vi "Enum from Ring String.vi"(8 "String to Match":string, 9 "Ring Strings []":string[](array[string]), 11 "Ring StringsAndValues[]":T1) -> (0 "error out":errorcluster, 3 "Enum Value":i32)   [LabVIEW 2024]
uses:
  <vilib>/Utility/miscctls.llb/LVStringsAndValuesArrayTypeDef_I32.ctl
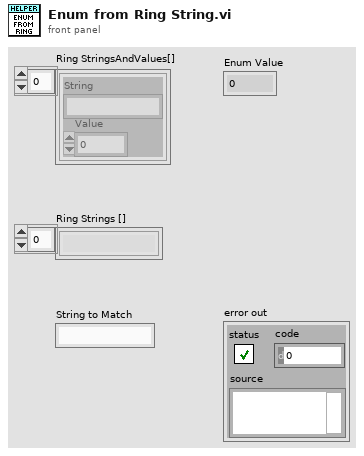
[diagram p1: front panel]
types:
  T1 = typedef "LVStringsAndValuesArrayTypeDef_I32.ctl" = cluster{"String":string, "Value":i32}[]
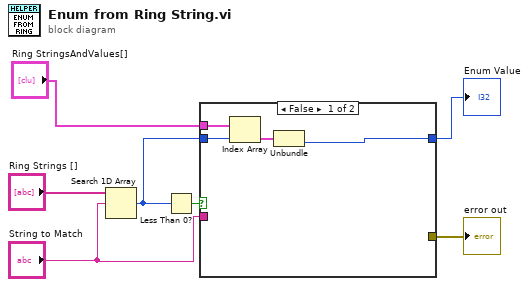
[diagram p0: block diagram]
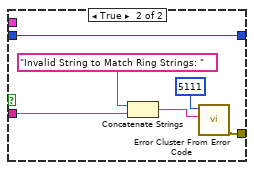
[diagram p2: hidden frame]
diagram:
  n1 = Search 1D Array(1D array="Ring Strings []", element="String to Match") -> (index of element=w2:i32)  [unwired: 1 in]
  n2 = Less Than 0?(x=w2) -> (x < 0?=w4:bool)
  n3 = case shown="False" w4 {
    tunnel: [_ w16] -> w6
    tunnel: "String to Match" -> [_ w14]
    tunnel: "Ring StringsAndValues[]" -> [w10 _]
    tunnel: w2 -> [w9 w12]
    tunnel: [w8 w12] -> w1
    frame False {
      n4 = Index Array(array=w10, index=w9) -> (element=w11:cluster{"String":string, "Value":i32})
      n5 = Unbundle(w11) -> ("Value"=w8:i32)  [unwired: 1 out]
    }
    frame True {
      n6 = Concatenate Strings("Invalid String to Match Ring Strings: " ("string"), w14) -> (w13:string)
      n7 = call <vilib>:"Error Cluster From Error Code.vi"("error message (\"\")"=w13, "error code (0)"=5111) -> ("error out"=w16:errorcluster)  [unwired: 7 in]
    }
  }
  "Enum Value" <- w1
  "error out" <- w6
